vi "Orion PDU Test Program.vi"(8 "error in (no error)":errorcluster) -> (0 "error out":errorcluster)   [LabVIEW 2024]
uses:
  <vilib>/httpClient/POSTBuffer.vi
  <vilib>/httpClient/LabVIEWHTTPClient.lvlib
panel:
  out "body":string
  out "headers":string
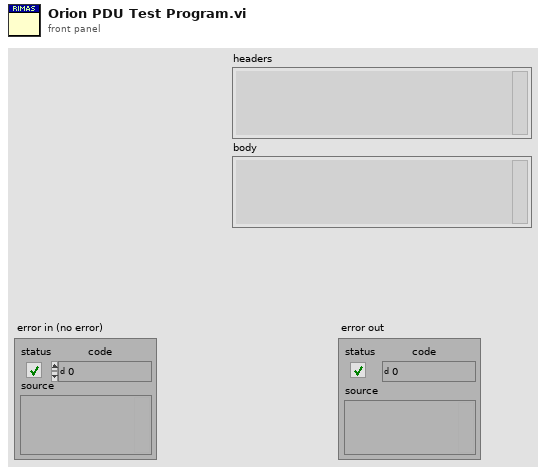
[diagram p1: front panel]
types:
  T1 = typedef "LabVIEWHTTPClient.lvlib/ClientHandle.ctl" = refnum<k1>
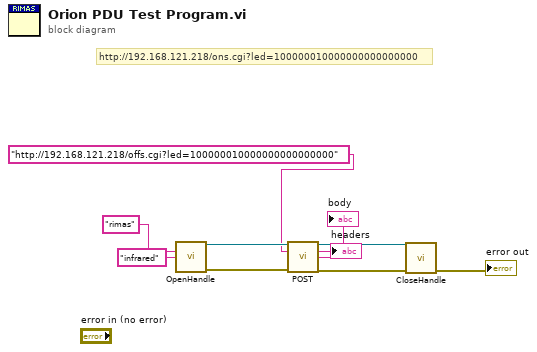
[diagram p0: block diagram]
diagram:
  # "http://192.168.121.218/ons.cgi?led=100000010000000000000000"
  n1 = call <vilib>:"OpenHandle.vi"("username"="rimas", "password"="infrared") -> ("client handle out"=w10:T1, "error out"=w6:errorcluster)  [unwired: 12 in]
  n2 = call-poly <vilib>:"POST.vi"("client handle"=w10, "url"="http://192.168.121.218/offs.cgi?led=100000010000000000000000", "error in (no error)"=w6) -> ("client handle out"=w8:T1, "headers"=→"headers":string, "body"=→"body":string, "error out"=w7:errorcluster)  [unwired: 9 in]
  n3 = call <vilib>:"CloseHandle.vi"("client handle"=w8, "error in (no error)"=w7) -> ("error out"=→"error out":errorcluster)  [unwired: 13 in]
